vi "Initialize AI.vi"(8 "error in":errorcluster, 9 "samples per channel":i32=1000, 10 "rate":dbl=1000.0 format="%0.2f", 11 "Channels":string="ai0") -> (0 "error out":errorcluster, 3 "task out":refnum<k21>)   [LabVIEW 2023, in "AI.lvlib"]
uses:
  AI.lvlib
  <vilib>/DAQmx/create/channels.llb/DAQmx Create Channel (AI-Voltage-Basic).vi
  <vilib>/DAQmx/configure/timing.llb/DAQmx Timing (Sample Clock).vi
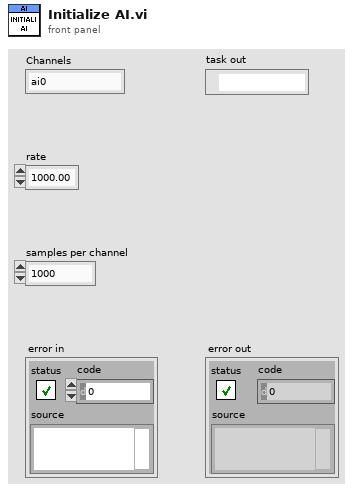
[diagram p1: front panel]
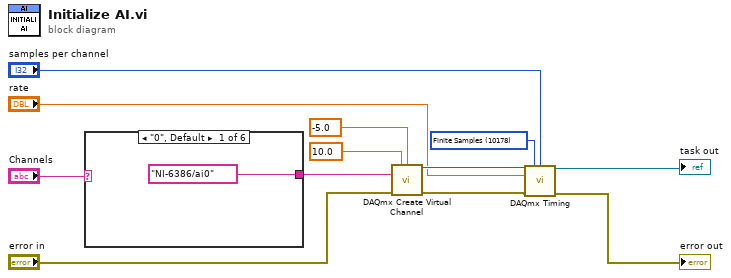
[diagram p0: block diagram]
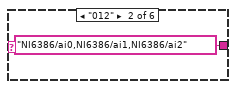
[diagram p2: hidden frame]
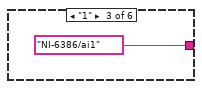
[diagram p3: hidden frame]
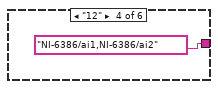
[diagram p4: hidden frame]
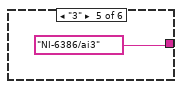
[diagram p5: hidden frame]
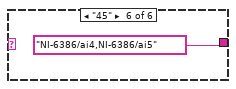
[diagram p6: hidden frame]
diagram:
  w4 = 10178 items=["Finite Samples"=10178, "Continuous Samples"=10123, "Hardware Timed Single Point"=12522] ("sample mode")
  n1 = case shown="\"0\", Default" "Channels" {
    tunnel: [tag "NI-6386/ai0" ("physical channels 3") tag "NI6386/ai0,NI6386/ai1,NI6386/ai2" ("physical channels 3") tag "NI-6386/ai1" ("physical channels 3") tag "NI-6386/ai1,NI-6386/ai2" ("physical channels 3") tag "NI-6386/ai3" ("physical channels 3") tag "NI-6386/ai4,NI-6386/ai5" ("physical channels 3")] -> w11
    frame "0", Default {
    }
    frame "012" {
    }
    frame "1" {
    }
    frame "12" {
    }
    frame "3" {
    }
    frame "45" {
    }
  }
  n2 = call-poly <vilib>:"DAQmx Create Virtual Channel.vi"("maximum value"=10.0, "minimum value"=-5.0, "physical channels"=w11, "error in"="error in") -> ("task out"=w8:refnum<k21>, "error out"=w6:errorcluster)  [unwired: 10 in]
  n3 = call-poly <vilib>:"DAQmx Timing.vi"("task/channels in"=w8, "sample mode"=w4, "samples per channel"="samples per channel", "rate"="rate", "error in"=w6) -> ("task out"=→"task out":refnum<k21>, "error out"=→"error out":errorcluster)  [unwired: 9 in]
